vi "GetNextStepsToExecute.vi"(8 "error in (no error)":errorcluster, 10 "beautify JSON?":bool=TRUE, 11 "SequenceManager in":refnum<class "SequenceManager.lvclass">) -> (0 "error out":errorcluster, 1 "Empty Array?":bool, 2 "Steps":refnum<class "Step.lvclass">[](array[class]), 3 "SequenceManager out":refnum<class "SequenceManager.lvclass">)   [LabVIEW 2023, in "Easy.SequenceManagerLabVIEW.lvlib" / "SequenceManager.lvclass"]
uses:
  SequenceManager.lvclass
  SequenceManager.lvclass/SequenceManager.ctl
  C:/Projects/Cutiss/SequenceManager/SequenceManager/LabViewWrapper/build/Easy.SequenceManager.dll
  build/Easy.SequenceManager.dll
  Step/Step.lvclass
panel:
  # "Connector Pane"
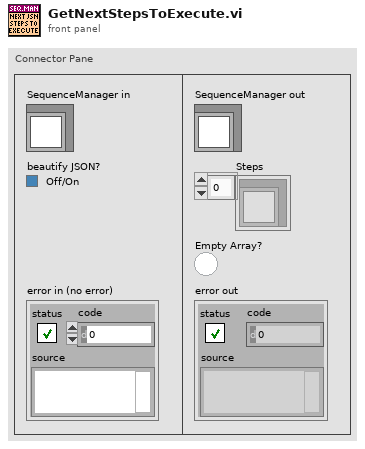
[diagram p1: front panel]
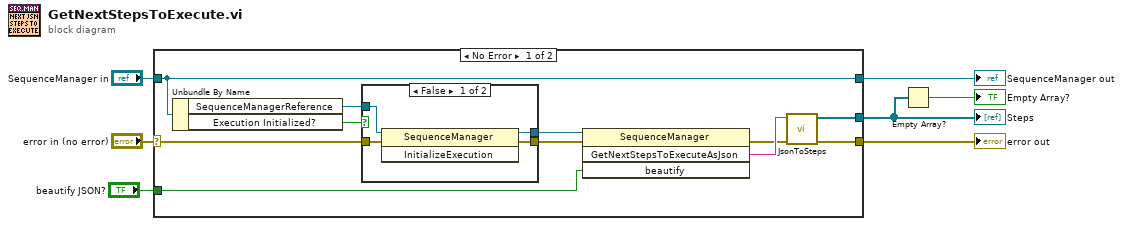
[diagram p0: block diagram]
diagram:
  n1 = case shown="No Error" "error in (no error)" {
    selector: "error in (no error)" -> [w15 w26]
    tunnel: [w8 w26] -> w6
    tunnel: [w18 w25] -> w4
    tunnel: "SequenceManager in" -> [w18 w25]
    tunnel: "beautify JSON?" -> [w12 _]
    tunnel: [w10 _] -> w1
    frame No Error {
      n2 = Unbundle By Name(w18) -> ("SequenceManagerReference"=w16:refnum<k24>, "Execution Initialized?"=w17:bool)
      n3 = case shown="False" w17 {
        tunnel: w16 -> [w21 w24]
        tunnel: [w20 w24] -> w14
        tunnel: w15 -> [w22 w23]
        tunnel: [w19 w23] -> w13
        frame False {
          n4 = invoke class="SequenceManager" method="InitializeExecution"(reference=w21, error in=w22) -> (reference out=w20:refnum<k24>, error out=w19:errorcluster)  [unwired: 1 in, 1 out]
        }
        frame True {
        }
      }
      n5 = invoke class="SequenceManager" method="GetNextStepsToExecuteAsJson"(reference=w14, error in=w13, "beautify"=w12) -> (error out=w9:errorcluster, "GetNextStepsToExecuteAsJson"=w11:string)  [unwired: 1 in, 2 out]
      n6 = call "JsonToSteps.vi"("error in (no error)"=w9, "JSON String"=w11) -> ("error out"=w8:errorcluster, "Steps"=w10:refnum<class "Step.lvclass">[])  [unwired: 8 in]
    }
    frame Error {
    }
  }
  "error out" <- w6
  "SequenceManager out" <- w4
  "Steps" <- w1
  n7 = Empty Array?(array=w1) -> (empty?=→"Empty Array?":bool)
